vi "ExpInitEnv.vi"(8 "error in (no error)":errorcluster, 10 "Enviroment path":path, 11 "Requires Matlab Enviroment":bool=TRUE) -> (0 "error out":errorcluster)   [LabVIEW 2017]
uses:
  ExpGlobals.vi
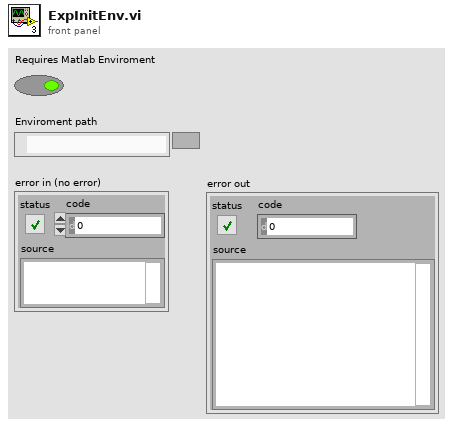
[diagram p1: front panel]
types:
  T1 = enum32{"Invalid", "Standard", "Closed", "Hidden", "Minimized", "Maximized"}
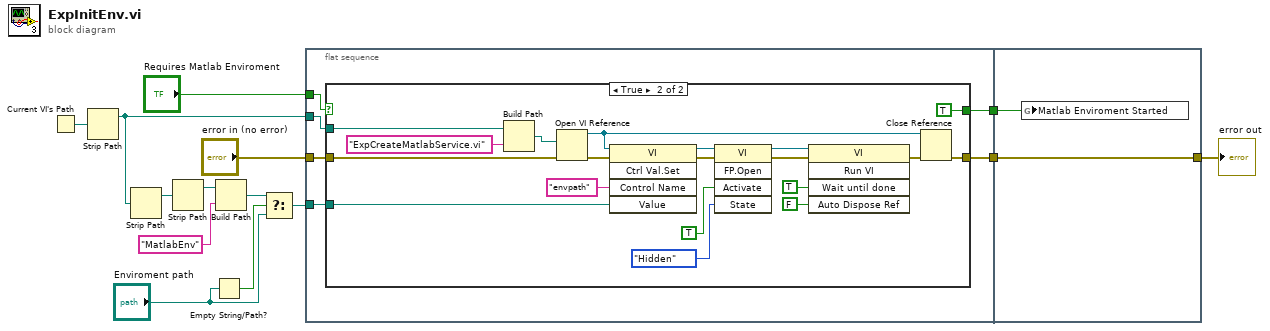
[diagram p0: block diagram]
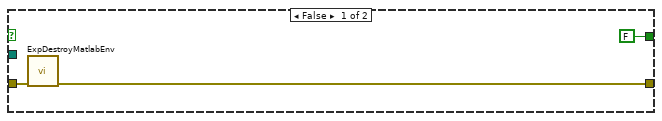
[diagram p2: hidden frame]
diagram:
  n1 = Current VI's Path() -> (path=w12:path)
  n2 = Strip Path(path=w12) -> (stripped path=w4:path)  [unwired: 1 out]
  n3 = Strip Path(path=w4) -> (stripped path=w11:path)  [unwired: 1 out]
  n4 = Strip Path(path=w11) -> (stripped path=w10:path)  [unwired: 1 out]
  n5 = Empty String/Path?(string/path="Enviroment path") -> (empty?=w14:bool)
  n6 = Build Path(base path=w10, name or relative path="MatlabEnv") -> (appended path=w8:path)
  n7 = Select(t=w8, s=w14, f="Enviroment path") -> (s? t:f=w7:path)
  n8 = flat-sequence {
    tunnel: w7 -> [w20]
    tunnel: "Requires Matlab Enviroment" -> [w19]
    tunnel: w4 -> [w17]
    tunnel: "error in (no error)" -> [w16]
    tunnel: [w18] -> w2
    tunnel: [w15] -> w1
    tunnel: [w44] -> w5
    tunnel: w2 -> [w44]
    tunnel: w1 -> [w43]
    frame #0 {
      n9 = case shown="True" w19 {
        tunnel: w20 -> [_ w39]
        tunnel: [w23 w31] -> w18
        tunnel: w17 -> [_ w28]
        tunnel: w16 -> [w22 w27]
        tunnel: [FALSE ("Matlab Enviroment Started") TRUE ("Matlab Enviroment Started")] -> w15
        frame False {
          n10 = call "ExpDestroyMatlabEnv.vi"("error in (no error)"=w22) -> ("error out"=w23:errorcluster)  [unwired: 10 in]
        }
        frame True {
          n11 = Build Path(base path=w28, name or relative path="ExpCreateMatlabService.vi") -> (appended path=w30:path)
          n12 = Open VI Reference(vi path=w30, error in (no error)=w27) -> (vi reference=w25:refnum<vi>, error out=w26:errorcluster)  [unwired: 4 in]
          n13 = invoke class="VI" method="Ctrl Val.Set"(reference=w25, error in=w26, "Control Name"="envpath", "Value"=w39) -> (reference out=w36:refnum<vi>, error out=w35:errorcluster)  [unwired: 1 in, 3 out]
          n14 = invoke class="VI" method="FP.Open"(reference=w36, error in=w35, "Activate"=TRUE ("Activate?"), "State"=T1."Hidden") -> (reference out=w34:refnum<vi>, error out=w33:errorcluster)  [unwired: 1 in, 3 out]
          n15 = invoke class="VI" method="Run VI"(reference=w34, error in=w33, "Wait until done"=TRUE ("Wait Until Done"), "Auto Dispose Ref"=FALSE ("Auto Dispose Reference")) -> (error out=w32:errorcluster)  [unwired: 1 in, 4 out]
          n16 = Close Reference(reference=w25, error in (no error)=w32) -> (error out=w31:errorcluster)
        }
      }
    }
    frame #1 {
      n17 = global write "ExpGlobals.vi" "Matlab Enviroment Started"(w43) -> ()
    }
  }
  "error out" <- w5
